vi "CurateFilesDelete.vi"() -> ()   [LabVIEW 2022 SP3]
panel:
  in  "length":i32
  out "Array 2":i32[](array[numeric])
  out "path out":path
  out "Array":path[](array[path])
  in  "index":i32
  in  "Boolean":bool
  out "size(s)":i32
  in  "Choose Directory":path=path "\\\\vantage-n-wk\\Vantage Data/Adam Doppler/2016-08-12/HFR_03A_20D_08kHz_16MHz_00_EYE"
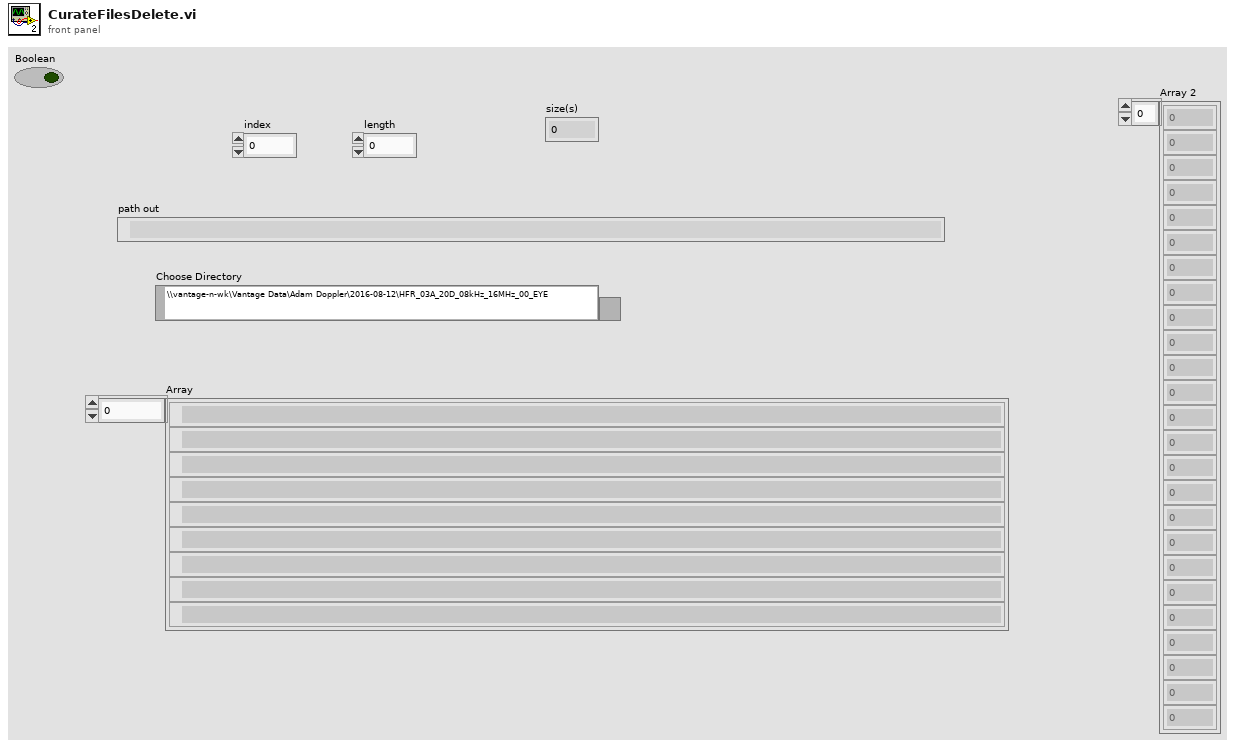
[diagram p1: front panel]
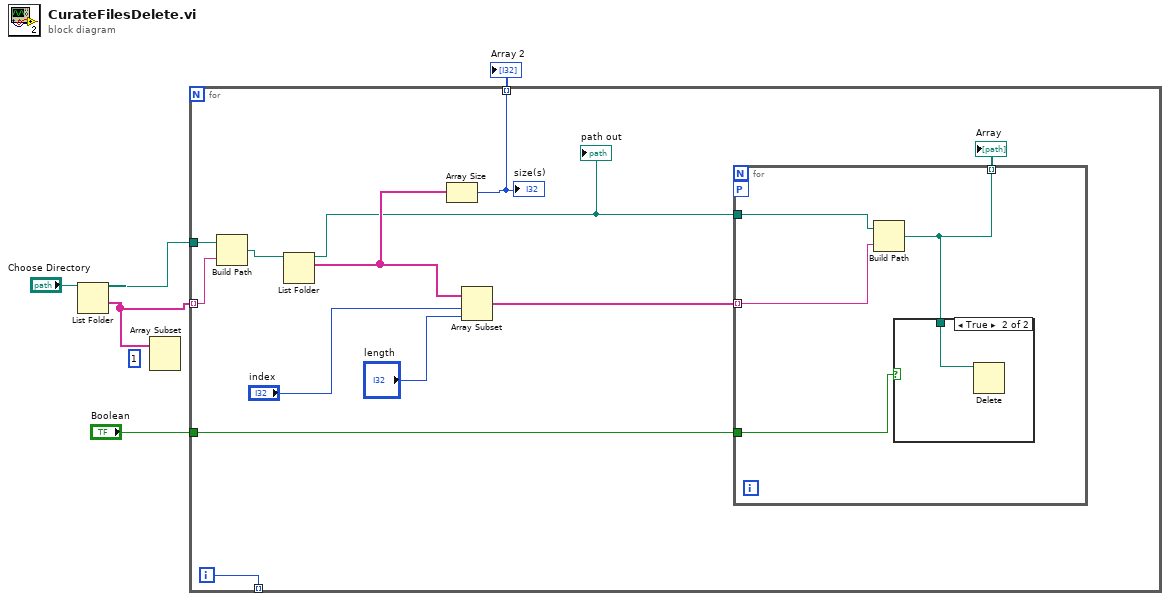
[diagram p0: block diagram]
diagram:
  (unwired) 1 ("index")
  n1 = List Folder(path="Choose Directory") -> (path out=w4:path, folder names=w1:string[])  [unwired: 2 in, 3 out]
  n2 = Array Subset(array=w1) -> ()  [unwired: 2 in, 1 out]
  n3 = for {
    tunnel: w1 -> [w14] mode=indexing
    tunnel: w4 -> [w13]
    tunnel: [w10] -> _ mode=indexing
    tunnel: "Boolean" -> [w9]
    tunnel: [w8] -> w2 mode=indexing
    i -> [w10]
    n4 = Build Path(base path=w13, name or relative path=w14) -> (appended path=w12:path)
    n5 = List Folder(path=w12) -> (path out=w15:path, filenames=w17:string[])  [unwired: 2 in, 3 out]
    "path out" <- w15
    n6 = Array Size(array=w17) -> (size(s)=w8:i32)
    "size(s)" <- w8
    n7 = Array Subset(array=w17, index="index", length="length") -> (w16:string[])
    n8 = for {
      tunnel: w16 -> [w21] mode=indexing
      tunnel: w15 -> [w20]
      tunnel: [w19] -> w11 mode=indexing
      tunnel: w9 -> [w18]
      workers-P: _ -> [_]
      n9 = Build Path(base path=w20, name or relative path=w21) -> (appended path=w19:path)
      n10 = case shown="True" w18 {
        tunnel: w19 -> [_ w22]
        frame False {
        }
        frame True {
          n11 = Delete(path (use dialog)=w22) -> ()  [unwired: 4 in, 3 out]
        }
      }
    }
    "Array" <- w11
  }
  "Array 2" <- w2
